vi "Read Drive Velocity High Gear.vi"(8 "error in (no error)":errorcluster, 11 "Drive in":refnum<class "Drive.lvclass">) -> (0 "error out":errorcluster, 2 "Slot":T1={"P"=0.0, "I"=0.0, "D"=0.0, "F"=0.0, "integralZone"=0.0, "allowableClosedLoopError"=0, "maxIntegralAccumulator"=0.0, "closedLoopPeakOutput"=1.0, "closedLoopPeriod"=1}, 3 "Drive out":refnum<class "Drive.lvclass">)   [LabVIEW 2018, in "Drive.lvlib" / "Drive.lvclass"]
uses:
  Drive.lvclass
  <vilib>/Rock Robotics/WPI/ThirdParty/Phoenix-LabVIEW/Motor Controller/Controls/CTRE_Phoenix_MotorControl_SlotStructure.ctl
  Drive.lvclass/Drive.ctl
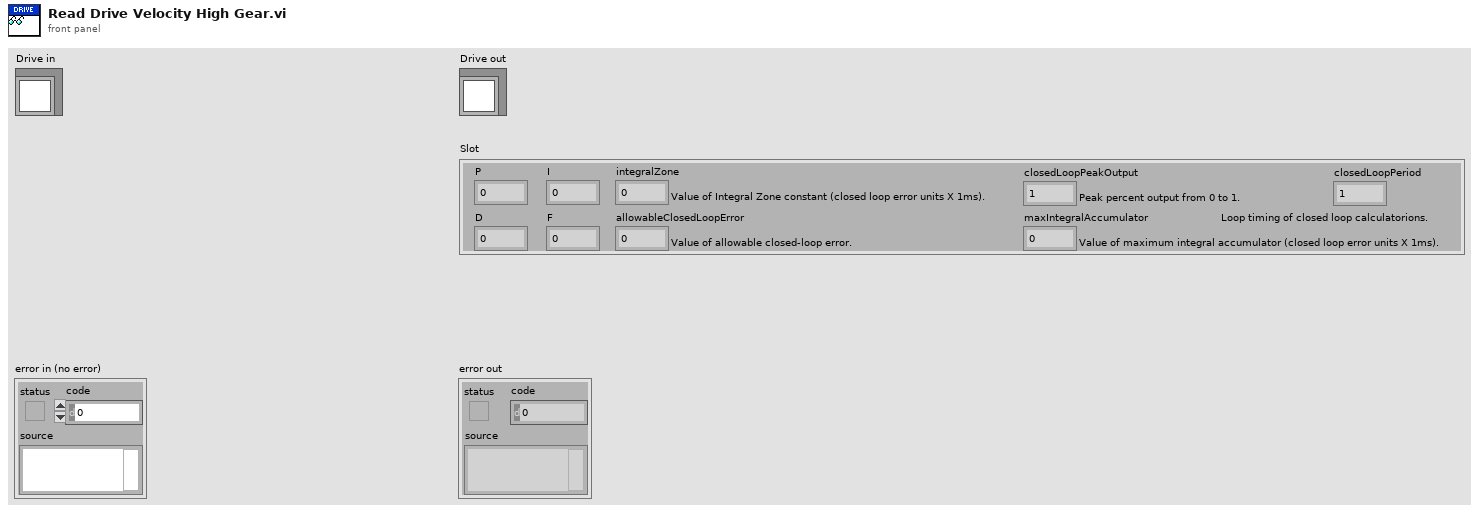
[diagram p1: front panel]
types:
  T1 = typedef "CTRE_Phoenix_MotorControl_SlotStructure.ctl" = cluster{"P":dbl, "I":dbl, "D":dbl, "F":dbl, "integralZone":dbl, "allowableClosedLoopError":i32, "maxIntegralAccumulator":dbl, "closedLoopPeakOutput":dbl, "closedLoopPeriod":i32}
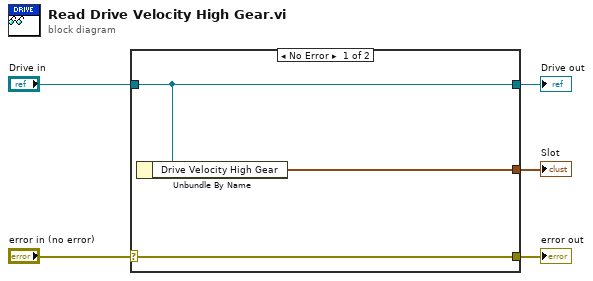
[diagram p0: block diagram]
diagram:
  n1 = case shown="No Error" "error in (no error)" {
    selector: "error in (no error)" -> [w8 w9]
    tunnel: [w8 w9] -> w4
    tunnel: [w7 w10] -> w2
    tunnel: "Drive in" -> [w7 w10]
    tunnel: [w6 _] -> w1
    frame No Error {
      n2 = Unbundle By Name(w7) -> ("Drive Velocity High Gear"=w6:T1)
    }
    frame Error {
    }
  }
  "error out" <- w4
  "Drive out" <- w2
  "Slot" <- w1
